vi "Set Element.vi"(8 "error in (no error)":errorcluster caption="entrée d'erreur (pas d'erreur)", 9 "variant":variant, 10 "nom":string, 11 "Container en entrée":refnum<class "Container.lvclass">) -> (0 "error out":errorcluster caption="sortie d'erreur", 3 "Container en sortie":refnum<class "Container.lvclass">)   [LabVIEW 2015, in "Container.lvclass"]
uses:
  Container.lvclass
  Container.lvclass/Container.ctl
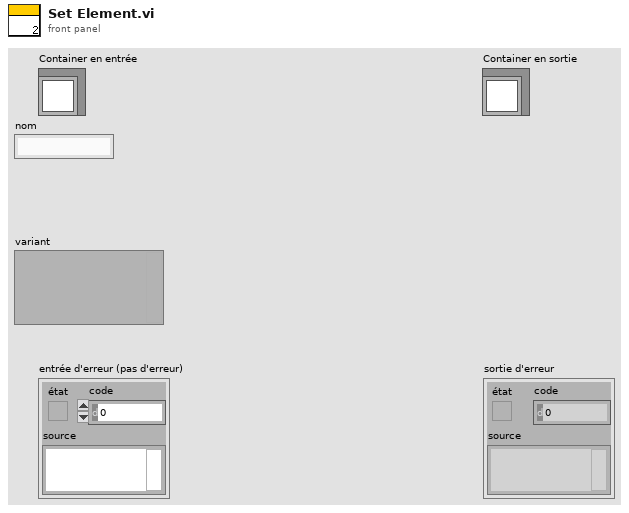
[diagram p1: front panel]
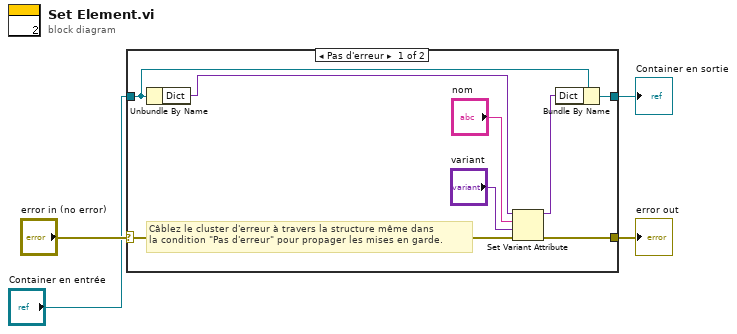
[diagram p0: block diagram]
diagram:
  n1 = case shown="Pas d'erreur" "error in (no error)" {
    selector: "error in (no error)" -> [w6 w14]
    tunnel: [w5 w14] -> w3
    tunnel: [w9 w13] -> w1
    tunnel: "Container en entrée" -> [w10 w13]
    frame No Error {
      # "Câblez le cluster d'erreur à travers la structure même dans\nla condition \"Pas d'erreur\" pour propager les mises en garde."
      n2 = Unbundle By Name(w10) -> ("Dict"=w12:variant)
      n3 = Set Variant Attribute(Variant=w12, name="nom", value="variant", error in=w6) -> (Variant out=w11:variant, error out=w5:errorcluster)  [unwired: 1 out]
      n4 = Bundle By Name(cluster=w10, "Dict"=w11) -> (w9:refnum<class "Container.lvclass">)
    }
    frame Error {
    }
  }
  "error out" <- w3
  "Container en sortie" <- w1
